vi "DTC.Export.vi"(8 "error in (no error)":errorcluster, 11 "Section Ref in":T1 format="%.0x") -> (0 "error out":errorcluster, 2 "DTC":T2 {"DTC Control"."Signals"."Byte Order" items=["Little Endian", "Big Endian"]; "DTC Control"."Signals"."Data Type" items=["Signed", "Unsigned", "IEEE Float"]}, 3 "Section Ref out":T1 format="%.0x")   [LabVIEW 2015, in "Diagnostics Addon System Explorer.lvlib"]
uses:
  Diagnostics Addon System Explorer.lvlib
  Types/DTC.Export.ctl
  Shared/Types/DTCDescriptor.ctl
  Types/DTCControl.Export.ctl
  Shared/Types/Signal.ctl
  <vilib>/NI Veristand/Custom Device API/Custom Device Item Ref.ctl
  Types/FG.Action.ctl
  Signals.Get.vi
  Type.FG.vi
  Signal.FG.vi
  <vilib>/NI Veristand/Custom Device API/NI VeriStand - Get Item Property.vi
  <vilib>/NI Veristand/Custom Device API/Get Item Property (U32).vi
  <vilib>/NI/NI VeriStand Advanced SysDef API/SysDef API/SysDef.Property.Set.vi
  <vilib>/NI/NI VeriStand Advanced SysDef API/_SubVIs/SysDef.Property.Set.U32.vi
  Shared/SubVIs/Constants.vi
  <vilib>/NI Veristand/Custom Device API/NI VeriStand - Get Custom Device Channel Data.vi
  <vilib>/NI Veristand/Custom Device API/Get Item Property (String).vi
  <vilib>/NI Veristand/Custom Device API/Get Item Property (Double).vi
  <vilib>/NI/NI VeriStand Advanced SysDef API/_SubVIs/SysDef.Property.Set.String.vi
  <vilib>/NI/NI VeriStand Advanced SysDef API/_SubVIs/SysDef.Property.Set.DBL.vi
  <vilib>/NI Veristand/Custom Device API/NI VeriStand - Get Item Children.vi
  <vilib>/NI Veristand/Custom Device Tools/Custom Device Utility Library/NI VeriStand - Search for Item by GUID.vi
  <vilib>/NI Veristand/Custom Device API/Get Item Property (String Array).vi
  <vilib>/NI Veristand/Custom Device API/Get Item Property (Double Array).vi
  <vilib>/NI Veristand/Custom Device API/Get Item Property (I32).vi
  <vilib>/NI/NI VeriStand Advanced SysDef API/_SubVIs/SysDef.Property.Set.String.Array.vi
  <vilib>/NI/NI VeriStand Advanced SysDef API/_SubVIs/SysDef.Property.Set.DBL.Array.vi
  <vilib>/NI/NI VeriStand Advanced SysDef API/_SubVIs/SysDef.Property.Set.I32.vi
  <vilib>/NI Veristand/Custom Device Tools/Custom Device Utility Library/NI VeriStand - Search for All Items by GUID.vi
  <vilib>/NI VeriStand/Custom Device Tools/Custom Device Utility Library/Custom Device Utility Library.lvlib
  <vilib>/NI VeriStand/Custom Device API/Custom Device API.lvlib
  Shared/Diagnostics Addon Shared.lvlib
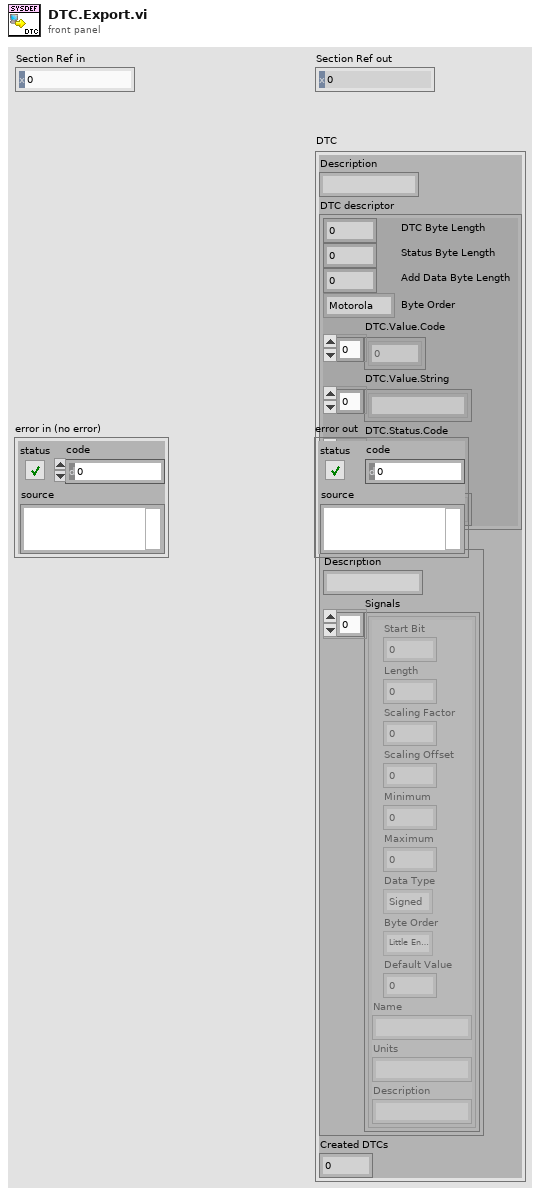
[diagram p1: front panel]
types:
  T1 = typedef "Custom Device API.lvlib/Custom Device Item Ref.ctl" = u64
  T2 = typedef "Diagnostics Addon System Explorer.lvlib/DTC.Export.ctl" = cluster{"Description":string, "DTC descriptor":T3, "DTC Control":T4, "Created DTCs":u32}
  T3 = typedef "Diagnostics Addon Shared.lvlib/DTCDescriptor.ctl" = cluster{"DTC Byte Length":i32, "Status Byte Length":i32, "Add Data Byte Length":i32, "Byte Order":enum16{"Motorola", "Intel"}, "DTC.Value.Code":dbl[], "DTC.Value.String":string[], "DTC.Status.Code":dbl[], "DTC.Status.String":string[]}
  T4 = typedef "Diagnostics Addon System Explorer.lvlib/DTCControl.Export.ctl" = cluster{"Description":string, "Signals":T5[]}
  T5 = typedef "Diagnostics Addon Shared.lvlib/Signal.ctl" = cluster{"Start Bit":u32, "Length":u32, "Scaling Factor":dbl, "Scaling Offset":dbl, "Minimum":dbl, "Maximum":dbl, "Data Type":u32, "Byte Order":u32, "Default Value":dbl, "Name":string, "Units":string, "Description":string}
  T6 = typedef "Diagnostics Addon System Explorer.lvlib/FG.Action.ctl" = enum16{"Get", "Set"}
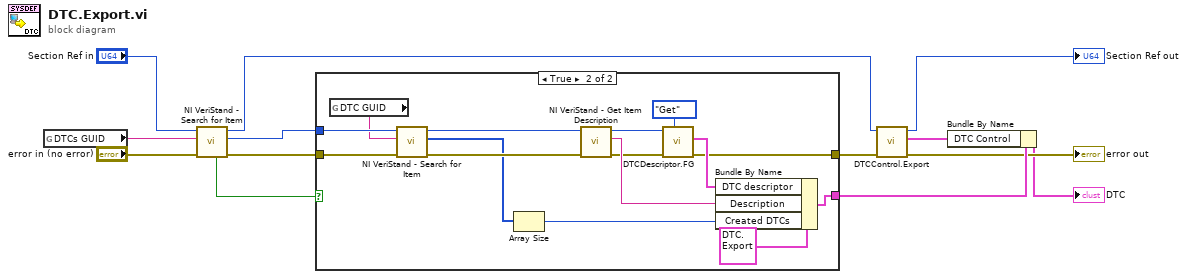
[diagram p0: block diagram]
diagram:
  n1 = global read "Constants.vi" "DTCs GUID"() -> (w8:string)
  n2 = call-poly <vilib>:"NI VeriStand - Search for Item.vi"("error in"="error in (no error)", "Item GUID"=w8, "Section Ref in"="Section Ref in") -> ("error out"=w11:errorcluster, "Item Ref"=w12:T1, "Section Ref out"=w4:T1, "Found"=w7:bool)  [unwired: 5 in]
  n3 = case shown="True" w7 {
    tunnel: [_ w29] -> w13
    tunnel: w12 -> [_ w19]
    tunnel: w11 -> [w14 w21]
    tunnel: [w14 w22] -> w6
    frame False {
    }
    frame True {
      n4 = global read "Constants.vi" "DTC GUID"() -> (w17:string)
      n5 = call-poly <vilib>:"NI VeriStand - Search for Item.vi"("error in"=w21, "Item GUID"=w17, "Section Ref in"=w19) -> ("error out"=w20:errorcluster, "Item Refs"=w16:T1[], "Section Ref out"=w18:T1)  [unwired: 5 in, 1 out]
      n6 = Array Size(array=w16) -> (size(s)=w15:i32)
      n7 = call <vilib>:"NI VeriStand - Get Item Description.vi"("error in (no error)"=w20, "Item Ref in"=w18) -> ("error out"=w24:errorcluster, "Description"=w27:string, "Item Ref out"=w25:T1)  [unwired: 7 out]
      n8 = call "DTCDescriptor.FG.vi"("Action"=FG.Action."Get", "error in (no error)"=w24, "Device Item Ref in"=w25) -> ("error out"=w22:errorcluster, "DTC descriptor"=w28:T3)  [unwired: 6 in, 1 out]
      n9 = Bundle By Name(cluster=T2 {"Description"="", "DTC descriptor"={"DTC Byte Length"=2, "Status Byte Length"=1, "Add Data Byte Length"=1, "Byte Order"=enum."Motorola", "DTC.Value.Code"=[], "DTC.Value.String"=[], "DTC.Status.Code"=[], "DTC.Status.String"=[]}, "DTC Control"={"Description"="", "Signals"=[]}, "Created DTCs"=0}, "DTC descriptor"=w28, "Description"=w27, "Created DTCs"=w15) -> (w29:T2)
    }
  }
  n10 = call "DTCControl.Export.vi"("error in (no error)"=w6, "Section Ref in"=w4) -> ("error out"=→"error out":errorcluster, "DTCControl"=w1:T4, "Section Ref out"=→"Section Ref out":T1)  [unwired: 7 in]
  n11 = Bundle By Name(cluster=w13, "DTC Control"=w1) -> (→"DTC":T2)
